vi "Setup.vi"(11 "Dev Panel in":refnum<class "Dev Panel.lvclass">) -> (0 "error out":errorcluster, 3 "Dev Panel out":refnum<class "Dev Panel.lvclass">)   [LabVIEW 2021, in "Dev Panel.lvclass"]
uses:
  Dev Panel.lvclass
  Dev Panel.lvclass/Dev Panel.ctl
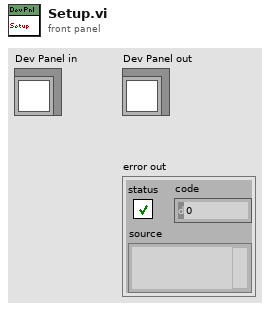
[diagram p1: front panel]
types:
  T1 = enum32{"Invalid", "Standard", "Closed", "Hidden", "Minimized", "Maximized"}
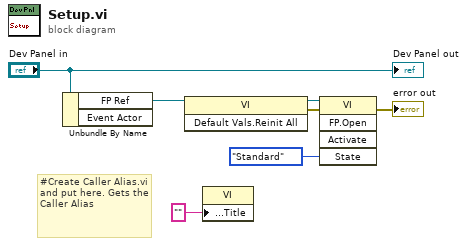
[diagram p0: block diagram]
diagram:
  # "#Create Caller Alias.vi\nand put here. Gets the Caller Alias"
  n1 = Unbundle By Name("Dev Panel in") -> ("FP Ref"=w2:refnum<vi>)  [unwired: 1 out]
  n2 = invoke class="VI" method="Default Vals.Reinit All"(reference=w2) -> (reference out=w3:refnum<vi>, error out=w4:errorcluster)  [unwired: 2 in, 1 out]
  n3 = property class="VI"("Front Panel.Title"="" ("Front Panel Window:Title")) -> ()  [unwired: 2 in, 2 out]
  n4 = invoke class="VI" method="FP.Open"(reference=w3, error in=w4, "State"=T1."Standard") -> (error out=→"error out":errorcluster)  [unwired: 2 in, 4 out]
  "Dev Panel out" <- "Dev Panel in"
